vi "dvp Vi Set Trigger Jitter Filter.vi"(10 "TriggerJitterFilter":dbl, 11 "handle":u32) -> (3 "function return":u32(ring))   [LabVIEW 2018, in "LabViewDVPCamera.lvlib"]
doc: "LabviewDvp2Api dvpStatus dvpViSetTriggerJitterFilter(dvpHandle handle, double TriggerJitterFilter);"
uses:
  LabViewDVPCamera.lvlib
  LabViewDVPCamera/LabViewDVPCamera.dll
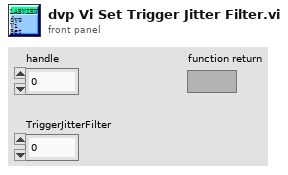
[diagram p1: front panel]
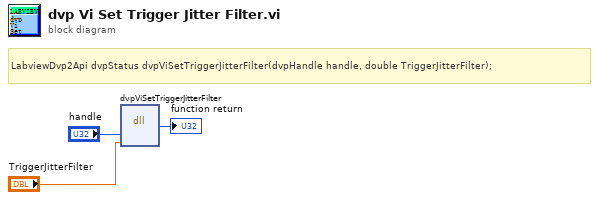
[diagram p0: block diagram]
diagram:
  # "LabviewDvp2Api dvpStatus dvpViSetTriggerJitterFilter(dvpHandle handle, double TriggerJitterFilter);"
  n1 = dll-call lib="C:/Program Files (x86)/DVP2 Labview cn 64/Sample/LabViewDVPCamera/LabViewDVPCamera.*" fn="dvpViSetTriggerJitterFilter"("handle"="handle", "TriggerJitterFilter"="TriggerJitterFilter") -> (→"function return":u32)  [unwired: 5 in, 2 out]
